vi "Log.vi"(8 "error":errorcluster, 10 "Msg":string, 11 "Log Level":T1) -> (0 "dup error":errorcluster)   [LabVIEW 2020, in "Logging.lvlib"]
uses:
  Logging.lvlib
  Define/Log Level.ctl
  Logger Mananger/Logger Mananger.lvclass
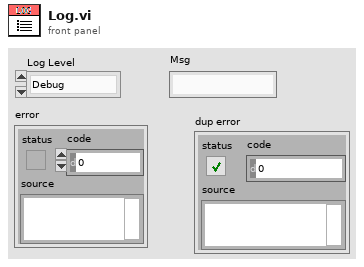
[diagram p1: front panel]
types:
  T1 = typedef "Logging.lvlib/Log Level.ctl" = enum16{"Debug", "Info", "Warn", "Error"}
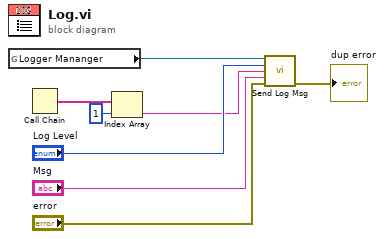
[diagram p0: block diagram]
diagram:
  n1 = global read "Global Log.vi" "Logger Mananger"() -> (w6:refnum<class "Logger Mananger.lvclass">)
  n2 = Call Chain() -> (call chain=w8:string[])
  n3 = Index Array(array=w8, index=1) -> (element=w4:string)
  n4 = call "Send Log Msg.vi"("Logger Mananger in"=w6, "Log Level"="Log Level", "Caller"=w4, "Msg"="Msg", "error in (no error)"="error") -> ("error out"=→"dup error":errorcluster)  [unwired: 9 in, 1 out]
